vi "Test Set Cell Value dbl.vi"(11 "Test Case In":refnum<class "Test Open Xml.lvclass">) -> (0 "error out":errorcluster, 3 "Test Case Out":refnum<class "Test Open Xml.lvclass">)   [LabVIEW 2020, in "Test Open Xml.lvclass"]
uses:
  Test Open Xml.lvclass
  <vilib>/Astemes/LUnit/Test Case.lvclass
  Source/Open Xml.lvlib
  f76079c9-ef62-41ac-a871-70fbb9772100.vi
  Source/Cell DataType.ctl
  515be3ce-b14c-461f-a887-ee26e19603ff.vi
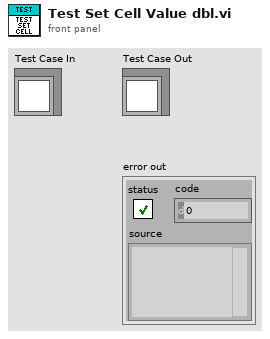
[diagram p1: front panel]
types:
  T1 = typedef "Open Xml.lvlib/Cell DataType.ctl" = enum16{"Void", "Boolean", "Number", "Error", "SharedString", "String", "InlineString", "Date"}
  T2 = cluster{"Number":dbl, "String":string, "Boolean":bool, "Timestamp":timestamp, "Error":errorcluster}
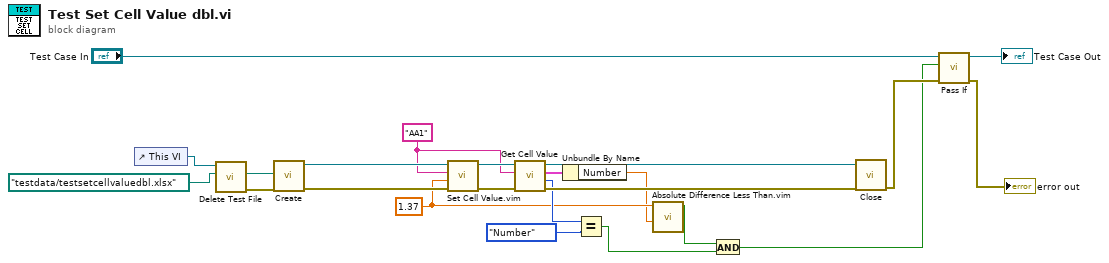
[diagram p0: block diagram]
diagram:
  w6 = 1.37
  w9 = "AA1" ("Cell Address")
  n1 = control-ref of="This VI"() -> (w16:refnum<vi>)
  n2 = call "Delete Test File.vi"("name or relative path"=path "testdata/testsetcellvaluedbl.xlsx", "VI in"=w16) -> ("error out"=w14:errorcluster, "deleted path"=w13:path)  [unwired: 8 in]
  n3 = call "Create.vi"("error in"=w14, "Path"=w13) -> ("error out"=w19:errorcluster, "SpreadsheetDoc"=w20:refnum<k24>)  [unwired: 8 in]
  n4 = call "Set Cell Value.vim"("error in"=w19, "Value"=w6, "Cell Address"=w9, "SpreadsheetDoc in"=w20) -> ("error out"=w12:errorcluster, "SpreadsheetDoc out"=w11:refnum<k24>)  [unwired: 6 in]
  n5 = call "Get Cell Value.vi"("error in"=w12, "Cell Address"=w9, "SpreadsheetDoc in"=w11) -> ("error out"=w10:errorcluster, "Type"=w8:T1, "Cell Value"=w5:T2, "SpreadsheetDoc out"=w17:refnum<k24>)  [unwired: 5 in]
  n6 = Unbundle By Name(w5) -> ("Number"=w1:dbl)
  n7 = Equal?(x=w8, y=Cell_DataType."Number") -> (x = y?=w4:bool)
  n8 = call "Absolute Difference Less Than.vim"("Number 2"=w1, "Number 1"=w6) -> ("In Limit"=w3:bool)  [unwired: 9 in]
  n9 = And(x=w3, y=w4) -> (x .and. y?=w2:bool)
  n10 = call "Close.vi"("error in"=w10, "SpreadsheetDoc"=w17) -> ("error out"=w18:errorcluster)  [unwired: 9 in]
  n11 = call <vilib>:"Pass If.vi"("error in (no error)"=w18, "Pass?"=w2, "LUnit Test Case In"="Test Case In") -> ("error out"=→"error out":errorcluster, "LUnit Test Case Out"=→"Test Case Out":refnum<class "Test Open Xml.lvclass">)  [unwired: 7 in]
